vi "Set Value.vi"(8 "error in (no error)":errorcluster, 10 "Variant":variant, 11 "Variant Value Source in":refnum<class "Variant Value Source.lvclass">) -> (0 "error out":errorcluster, 3 "Variant Value Source out":refnum<class "Variant Value Source.lvclass">)   [LabVIEW 2020, in "Composed Columns.lvlib" / "Variant Value Source.lvclass"]
uses:
  Variant Value Source.lvclass
  Variant Value Source.lvclass/Variant Value Source.ctl
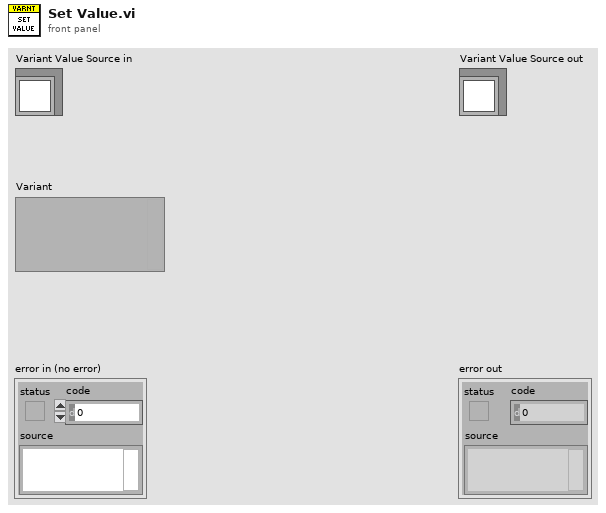
[diagram p1: front panel]
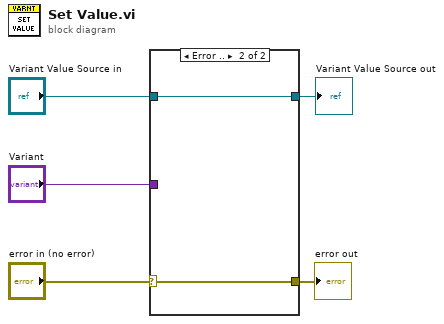
[diagram p0: block diagram]
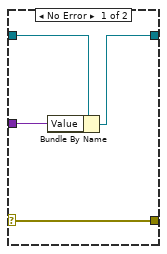
[diagram p2: hidden frame]
diagram:
  n1 = case shown="Error .." "error in (no error)" {
    selector: "error in (no error)" -> [w9 w10]
    tunnel: [w9 w10] -> w4
    tunnel: "Variant Value Source in" -> [w8 w11]
    tunnel: [w7 w11] -> w2
    tunnel: "Variant" -> [w6 _]
    frame No Error {
      n2 = Bundle By Name(cluster=w8, "Value"=w6) -> (w7:refnum<class "Variant Value Source.lvclass">)
    }
    frame Error {
    }
  }
  "error out" <- w4
  "Variant Value Source out" <- w2
